vi "Dispose.vi"(0 "Display State In":T1, 9 "Container State":T2, 11 "error in (no error)":errorcluster) -> (4 "Display State Out":T1, 15 "error out":errorcluster)   [LabVIEW 2020, in "WebView2 XControl.lvlib" / "WebView2 Control.xctl"]
uses:
  <vilib>/_xctls/Container State.ctl
  WebView2 Control.xctl
  Webview2 Lib/WebView2 Control Object/WebView2 Control.lvclass
  <vilib>/_xctls/XControlSupport.lvlib
  State.ctl
panel:
  # "Add Controls & Indicators that form the parameters of the method here. Hook them to the connector pane. Do not delete the controls & indicators that are already hooked to the connector pane.\n \nTo setup the parameters  for this method, right click on this item in the Project Tree & select \"Configure Method...\"."
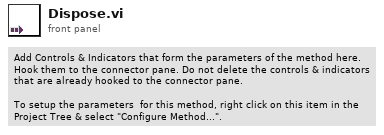
[diagram p1: front panel]
types:
  T1 = typedef "WebView2 XControl.lvlib/WebView2 Control.xctl/State.ctl" = cluster{"Control Object Ref":refnum<data-value>}
  T2 = typedef "XControlSupport.lvlib/Container State.ctl" = cluster{"Indicator?":bool, "Run Mode?":bool, " Refnum":refnum<vi>}
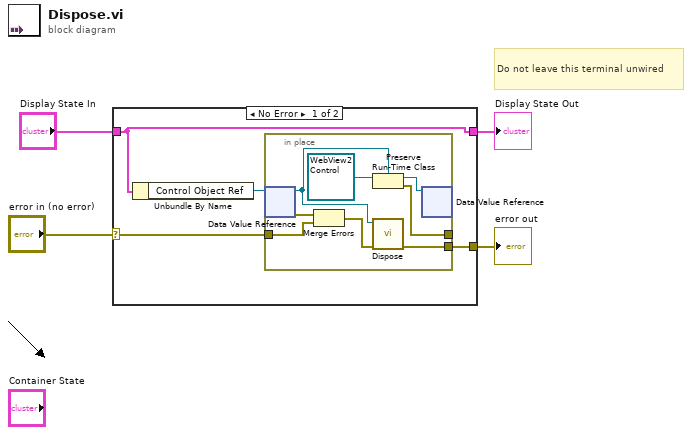
[diagram p0: block diagram]
diagram:
  # "Do not leave this terminal unwired"
  n1 = case shown="No Error" "error in (no error)" {
    selector: "error in (no error)" -> [w6 w18]
    tunnel: [w5 w18] -> w1
    tunnel: "Display State In" -> [w8 w17]
    tunnel: [w8 w17] -> w3
    frame No Error {
      n2 = Unbundle By Name(w8) -> ("Control Object Ref"=w7:refnum<data-value>)
      n3 = in-place {
        in-place-border: w6 -> [w14]
        in-place-border: [w13] -> w5
        in-place-border: [w9] -> _
        n4 = in-place-dvr #1(w7) -> (w11:refnum<class "WebView2 Control.lvclass">, w16:errorcluster)
        n5 = Merge Errors(w16, w14) -> (w15:errorcluster)
        n6 = Preserve Run-Time Class(object in=refnum<class "WebView2 Control.lvclass"> refnum, 2:w11) -> (object out=w12:refnum<class "WebView2 Control.lvclass">, error out=w9:errorcluster)  [unwired: 1 in]
        n7 = call "Dispose.vi"("error in (no error)"=w15, "WebView2 Control in"=w11) -> ("error out"=w13:errorcluster)  [unwired: 9 in]
        n8 = in-place-dvr #1(w12) -> ()  [unwired: 2 out]
      }
    }
    frame Error {
    }
  }
  "Display State Out" <- w3
  "error out" <- w1
